vi "启动多探头.vi"(11 "探头数量":i32=3) -> (3 "探头数量 o":i32)   [LabVIEW 2017]
panel:
  in  "标志-停止":bool
  in  "停止按钮":bool
  out "vi引用[]":refnum<vi>[](array[refnum])
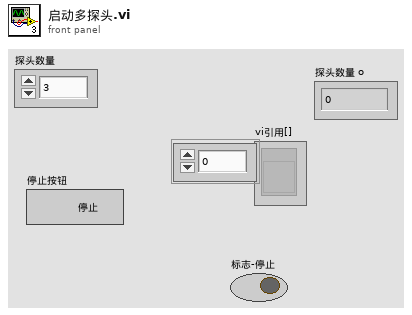
[diagram p1: front panel]
types:
  T1 = enum32{"Invalid", "Standard", "Closed", "Hidden", "Minimized", "Maximized"}
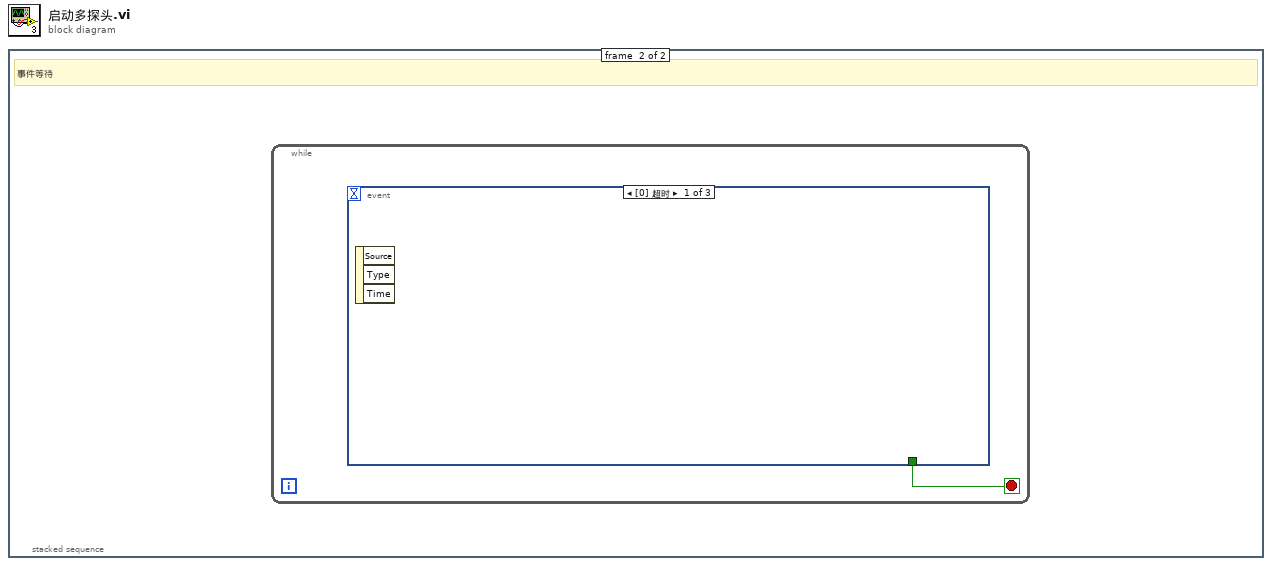
[diagram p0: block diagram]
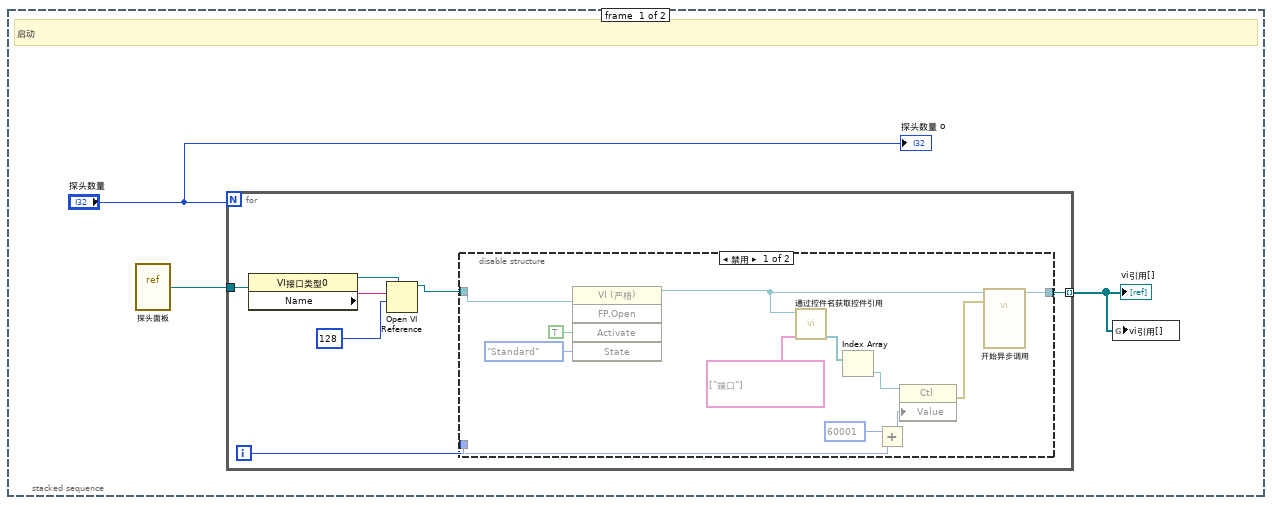
[diagram p2: hidden frame]
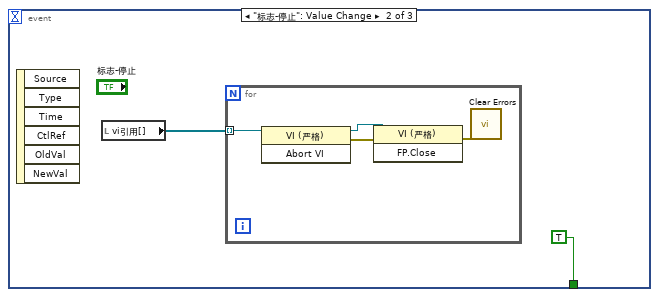
[diagram p4: hidden frame]
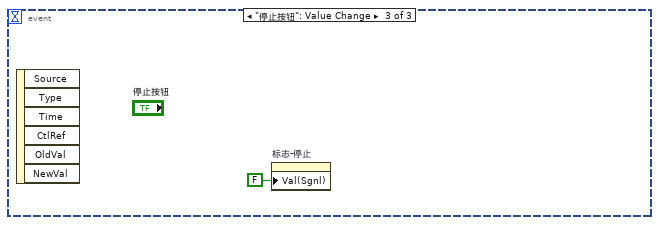
[diagram p5: hidden frame]
diagram:
  n1 = stacked-sequence {
    frame #0 {
      # "启动"
      n2 = vi-ref "探头面板.vi"() -> (w3:refnum<vi>)
      n3 = for {
        N: "探头数量" -> [_]
        tunnel: w3 -> [w10]
        tunnel: [w6] -> w1 mode=indexing
        i -> [w5]
        n4 = property class="VI接口类型0"(reference=w10) -> (reference out=w7:refnum<vi>, "Name"=w8:string)  [unwired: 1 in, 1 out]
        n5 = Open VI Reference(type specifier VI Refnum (for type only)=w7, vi path=w8, options=128 ("选项")) -> (vi reference=w4:refnum<vi>)  [unwired: 3 in, 1 out]
        n6 = disable-structure shown="禁用" {
          disable-tunnel: w4 -> [w11 w23]
          disable-tunnel: [w20 w23] -> w6
          disable-tunnel: w5 -> [w18 _]
          frame Disabled {
            n7 = invoke class="VI (严格)" method="FP.Open"(reference=w11, "Activate"=TRUE ("激活？"), "State"=T1."Standard" ("状态")) -> (reference out=w12:refnum<vi>)  [unwired: 2 in, 4 out]
            n8 = call "通过控件名获取控件引用.vi"("控件名数组"=string[] ["端口"], "VI引用"=w12) -> ("控件引用输出"=w22:refnum<vi>[])  [unwired: 7 in, 2 out]
            n9 = Index Array(array=w22) -> (element=w19:refnum<vi>)  [unwired: 1 in]
            n10 = Add(x=60001, y=w18) -> (x+y=w17:i32)
            n11 = property class="Ctl"(reference=w19, "Value"=w17) -> (error out=w15:errorcluster)  [unwired: 1 in, 1 out]
            n12 = call-by-ref "开始异步调用"(reference=w12, error in=w15) -> (reference out=w20:refnum<vi>)  [unwired: 12 in, 1 out]
          }
          frame Enabled {
          }
        }
      }
      "vi引用[]" <- w1
      n13 = global write "全局-模拟器变量.vi" "vi引用[]"(w1) -> ()
      "探头数量 o" <- "探头数量"
    }
    frame #1 {
      # "事件等待"
      n14 = while {
        stop <- w24 stop-if-true
        n15 = event shown="[0] 超时" {
          selector: _ -> [_ _ _]
          dyn-events: _ -> [_ _ _]
          timeout: _ -> [_ _ _]
          tunnel: [_ TRUE _] -> w24
          event Timeout {
            n16 = event-data() -> ()  [unwired: 1 in, 3 out]
          }
          event "标志-停止": Value Change {
            n17 = event-data() -> ()  [unwired: 1 in, 6 out]
            n18 = local read "vi引用[]"() -> (w25:refnum<vi>[])
            n19 = for {
              tunnel: w25 -> [w30] mode=indexing
              n20 = invoke class="VI (严格)" method="Abort VI"(reference=w30) -> (reference out=w29:refnum<vi>, error out=w28:errorcluster)  [unwired: 2 in, 1 out]
              n21 = invoke class="VI (严格)" method="FP.Close"(reference=w29, error in=w28) -> (error out=w27:errorcluster)  [unwired: 1 in, 2 out]
              n22 = call <vilib>:"Clear Errors.vi"("error in (no error)"=w27) -> ()  [unwired: 5 in, 2 out]
            }
          }
          event "停止按钮": Value Change {
            n23 = event-data() -> ()  [unwired: 1 in, 6 out]
            n24 = property on="标志-停止" class="Bool (严格)"("Val(Sgnl)"=FALSE ("值(信号)")) -> ()  [unwired: 2 in, 2 out]
          }
        }
      }
    }
  }
